vi "Global_SM Write_Data Out.vi"() -> ()   [LabVIEW 2017, in "Lift.lvlib"]
uses:
  Lift.lvlib
  _SHARE ALL/TypeDef Share All/CLUSTER_TalonInput.ctl
  _SHARE ALL/RoboRio Share All/SRX Share All/TypeDefs SRX/Cluster_SRX_PIDF.ctl
  _SHARE ALL/RoboRio Share All/SRX Share All/TypeDefs SRX/Cluster_SRX_Mode and Value.ctl
  System Drivers/Phoenix-LabVIEW/Motor Controller/Controls/CTRE_Phoenix_MotorControl_ControlMode.ctl
  ENUM_SM_State.ctl
panel:
  in  "Lift_SM_State":T1
  in  "Lift_SM_Output":T2 {"SRXSet"."Mode" items=["PercentOutput"=0, "Position"=1, "Velocity"=2, "Current"=3, "Follower"=5, "MotionProfile"=6, "MotionMagic"=7, "MotionMagicArc"=8, "MotionProfileArc"=10, "Disabled"=15]}
  # "The Names of the Data items in the Global Variable MUST describe who the Single Writer is\nNaming Convention of all Data Items is:   \nLib Name_Loop Name (SM or SEN or ACT)_Data Name\nExamples:\nDrive_ACT_X axis\nGameController_SEN_JoystickLeft\nHopper_SM_AgitatorSpeed"
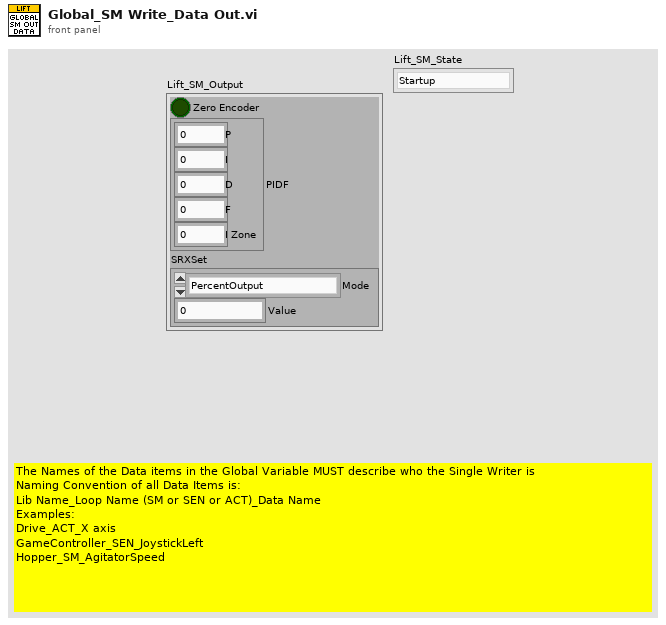
[diagram p1: front panel]
types:
  T1 = typedef "Lift.lvlib/ENUM_SM_State.ctl" = enum16{"Startup", "Idle", "F_Manual", "Manual", "Position - Moving", "Position - Holding", "Shutdown"}
  T2 = typedef "CLUSTER_TalonInput.ctl" = cluster{"Zero Encoder":bool, "PIDF":T3, "SRXSet":T4}
  T3 = typedef "Cluster_SRX_PIDF.ctl" = cluster{"P":dbl, "I":dbl, "D":dbl, "F":dbl, "I Zone":dbl}
  T4 = typedef "Cluster_SRX_Mode and Value.ctl" = cluster{"Mode":T5, "Value":dbl}
  T5 = typedef "CTRE_Phoenix_MotorControl_ControlMode.ctl" = u16
diagram:
